vi "GENERACION_REPORTE.vi"() -> ()   [LabVIEW 2021]
uses:
  <vilib>/Utility/NIReport.llb/Report Type.ctl
  <vilib>/Utility/NIReport.llb/Append Report Text (str wrap).vi
  <vilib>/Utility/NIReport.llb/NI_report.lvclass
  <vilib>/Utility/NIReport.llb/NI_ReportGenerationCore.lvlib
panel:
  in  "Save Button":bool
  out "new picture":picture
  in  "path to JPEG file":path
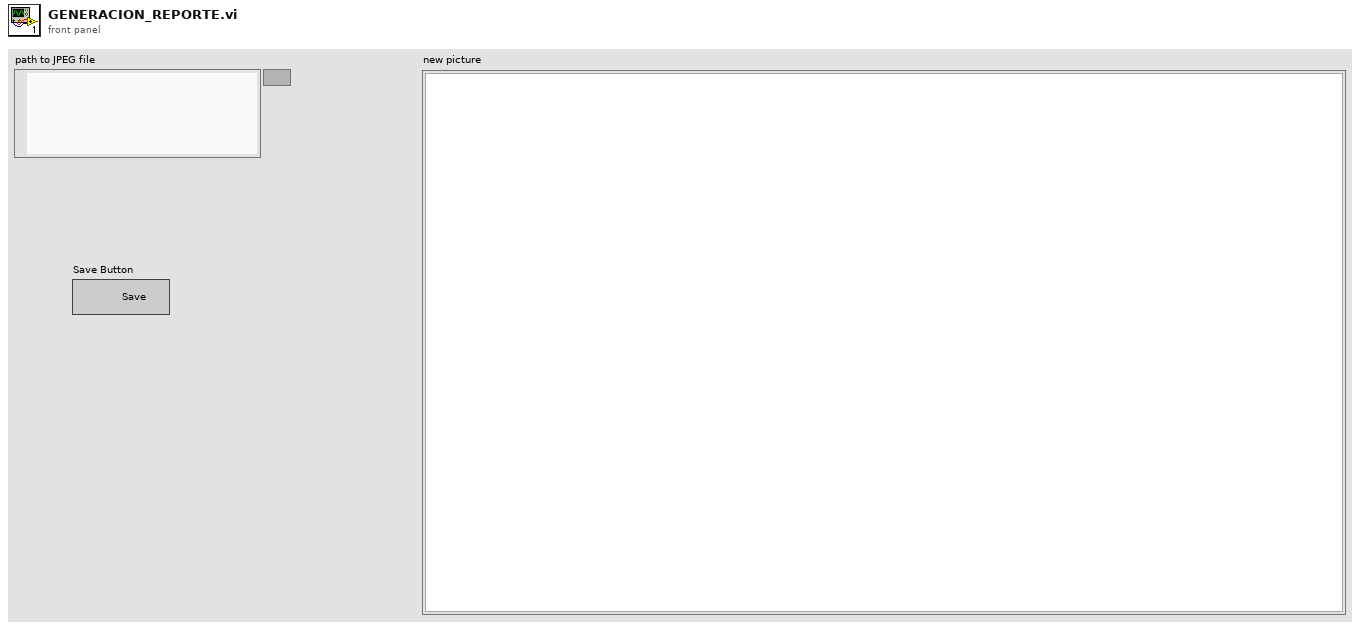
[diagram p1: front panel]
types:
  T1 = cluster{"Charset (-1)":i16, "Weight (-1)":i16, "Name":string, "Size":string}
  T2 = cluster{"Italic":enum16{"Italic Unchanged", "Italic On", "Italic Off"}, "Strike Through":enum16{"Strike Through Unchanged", "Strike Through On", "Strike Through Off"}, "Underline":enum16{"Underline Unchanged", "Underline On", "Underline Off"}, "Bold":enum16{"Bold Unchanged", "Bold On", "Bold Off"}}
  T3 = typedef "NI_ReportGenerationCore.lvlib/Report Type.ctl" = enum16{"HTML", "Word", "Excel"}
  T4 = typedef "imagedata.ctl" = cluster{"image type":i32, "image depth":i32, "image":u8[], "mask":u8[], "colors":u32[], "Rectangle":cluster{"left":i16, "top":i16, "right":i16, "bottom":i16}}
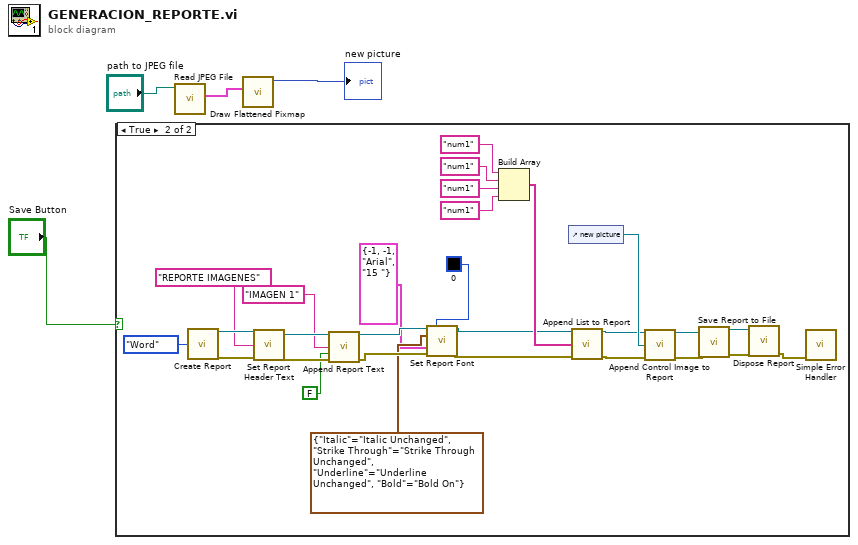
[diagram p0: block diagram]
diagram:
  n1 = case shown="True" "Save Button" {
    frame False {
    }
    frame True {
      n2 = call <vilib>:"Create Report.vi"("report type"=Report_Type."Word") -> ("report out"=w27:refnum<class "NI_report.lvclass">, "error out"=w26:errorcluster)  [unwired: 13 in]
      n3 = call-dynamic "Set Report Header Text.vi"("report in"=w27, "center header text"="REPORTE IMAGENES", "error in (no error)"=w26) -> ("report out"=w24:refnum<class "NI_report.lvclass">, "error out"=w23:errorcluster)  [unwired: 11 in]
      n4 = call-poly <vilib>:"Append Report Text.vi"("report in"=w24, "text"="IMAGEN 1", "append on new line? (F)"=FALSE, "error in (no error)"=w23) -> ("report out"=w20:refnum<class "NI_report.lvclass">, "error out"=w19:errorcluster)  [unwired: 8 in, 2 out]
      n5 = call-dynamic "Set Report Font.vi"("report in"=w20, "text color (unchanged)"=u32 0, "text options"=T2 {"Italic"=enum."Italic Unchanged", "Strike Through"=enum."Strike Through Unchanged", "Underline"=enum."Underline Unchanged", "Bold"=enum."Bold On"}, "font settings"=T1 {"Charset (-1)"=-1, "Weight (-1)"=-1, "Name"="Arial", "Size"="15 "}, "error in (no error)"=w19) -> ("report out"=w10:refnum<class "NI_report.lvclass">, "error out"=w9:errorcluster)  [unwired: 8 in, 1 out]
      n6 = Build Array("num1", "num1", "num1", "num1") -> (w11:string[])
      n7 = control-ref of="new picture"() -> (w8:refnum<vi>)
      n8 = call-dynamic "Append List to Report.vi"("report in"=w10, "list elements"=w11, "error in (no error)"=w9) -> ("report out"=w7:refnum<class "NI_report.lvclass">, "error out"=w6:errorcluster)  [unwired: 9 in, 2 out]
      n9 = call-dynamic "Append Control Image to Report.vi"("report in"=w7, "ctrl reference"=w8, "error in (no error)"=w6) -> ("report out"=w32:refnum<class "NI_report.lvclass">, "error out"=w31:errorcluster)  [unwired: 9 in, 2 out]
      n10 = call-dynamic "Save Report to File.vi"("report in"=w32, "error in (no error)"=w31) -> ("report out"=w30:refnum<class "NI_report.lvclass">, "error out"=w29:errorcluster)  [unwired: 12 in]
      n11 = call-dynamic "Dispose Report.vi"("report in"=w30, "error in (no error)"=w29) -> ("error out"=w5:errorcluster)  [unwired: 13 in]
      n12 = call <vilib>:"Simple Error Handler.vi"("error in (no error)"=w5) -> ()  [unwired: 4 in, 5 out]
    }
  }
  n13 = call <vilib>:"Read JPEG File.vi"("path to JPEG file"="path to JPEG file") -> ("image data"=w3:T4)  [unwired: 8 in, 2 out]
  n14 = call <vilib>:"Draw Flattened Pixmap.vi"("image data"=w3) -> ("new picture"=→"new picture":picture)  [unwired: 8 in]
